vi "Get TC Coefficients.vi"(11 "TC Inputs":string[][](array[string])) -> (1 "C":dbl, 2 "B":dbl, 3 "A":dbl)   [LabVIEW 2023, in "File Setup.lvlib"]
uses:
  File Setup.lvlib
  <vilib>/Analysis/NI_AALPro.lvlib
panel:
  out "Polynomial Coefficients":dbl[](array[numeric])
  out "array w/ subset deleted":string[][](array[string])
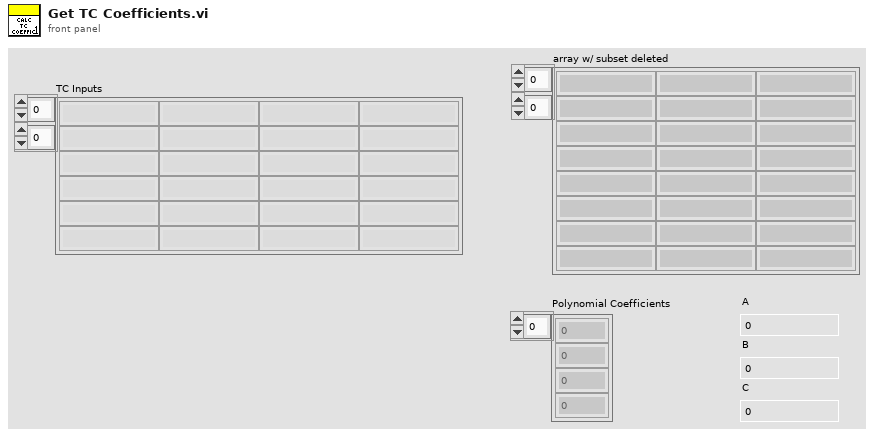
[diagram p1: front panel]
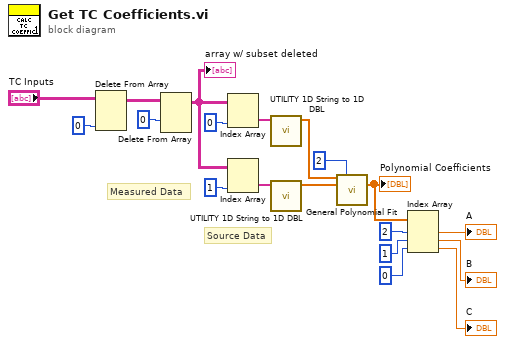
[diagram p0: block diagram]
diagram:
  # "Source Data"
  # "Measured Data"
  n1 = Delete From Array(array="TC Inputs", index (col)=0 ("disabled index (col)")) -> (array with subset deleted=w18:string[][])  [unwired: 2 in, 1 out]
  n2 = Delete From Array(array=w18, index (row)=0) -> (array with subset deleted=w14:string[][])  [unwired: 2 in, 1 out]
  "array w/ subset deleted" <- w14
  n3 = Index Array(array=w14, index (col)=0 ("disabled index (col)")) -> (element=w12:string[])  [unwired: 1 in]
  n4 = Index Array(array=w14, index (col)=1 ("disabled index (col)")) -> (element=w11:string[])  [unwired: 1 in]
  n5 = call "UTILITY 1D String to 1D DBL.vi"("Save Data"=w12) -> ("DBL"=w8:dbl[])  [unwired: 10 in]
  n6 = call "UTILITY 1D String to 1D DBL.vi"("Save Data"=w11) -> ("DBL"=w9:dbl[])  [unwired: 10 in]
  n7 = call <vilib>:"General Polynomial Fit.vi"("Y"=w8, "polynomial order"=2, "X"=w9) -> ("Polynomial Coefficients"=w7:dbl[])  [unwired: 9 in, 3 out]
  "Polynomial Coefficients" <- w7
  n8 = Index Array(array=w7, index #1=2 ("index"), index #2=1 ("index"), index #3=0 ("index")) -> (element #1=→"A":dbl, element #2=→"B":dbl, element #3=→"C":dbl)
